vi "Laser_COM.vi"() -> ()   [LabVIEW 2014]
uses:
  <vilib>/Instr/_visa.llb/Select Event Type.ctl
  <vilib>/Instr/_visa.llb/VISA Configure Serial Port (Instr).vi
panel:
  out "Laser":bool
  out "f, kHz":dbl caption="Темп. модуля" format="%#_g kHz"
  out "7":bool
  out "6":bool
  out "4":bool
  out "5":bool
  out "3":bool
  out "2":bool
  out "1":bool
  out "0":bool
  in  "Control PL":bool
  out "DB25 PL":bool
  out "RS232 PL":bool
  out "DB25 GL":bool
  out "RS232 GL":bool
  in  "Control GL":bool
  out "DB25 ML":bool
  out "RS232 ML":bool
  in  "Control ML":bool
  in  "Laser":bool
  out "Laser EM":bool caption="Излучение включено!"
  out "on/off? 3":bool
  out "on/off? 2":bool
  in  "Send":bool
  in  "write buffer":string caption="Передать команду"
  out "COM_connect":bool
  in  "Connect":bool
  out "SN:":string
  out "ID:":string
  out "Guide  laser":bool
  out "module temp":dbl caption="Темп. модуля" format="%#_g °C"
  in  "Power":dbl(slide) caption="Мощность излучения, %" min=0.0 max=100.0 step=0.5 scale=0.0..100.0 scale format="%#.2g"
  in  "Laser pilot":bool caption="Лазер пилот"
  in  "COM":refnum<visa-resource-name>="COM1" caption="Laser COM-port"
  out "read buffer":string caption="ОТВЕТ:"
  out "error out":errorcluster
  in  "error in (no error)":errorcluster
  # "ID:\n\nSN:"
  # "Блок  управления основным лазером"
  # "RS-232"
  # "DB-25"
  # "T модуля -"
  # "RS-232"
  # "Мощьность  излучения, %"
  # "DB-25"
  # "DB-25"
  # "Пилот Лазер"
  # "RS-232"
  # "DB-25"
  # "Терминал"
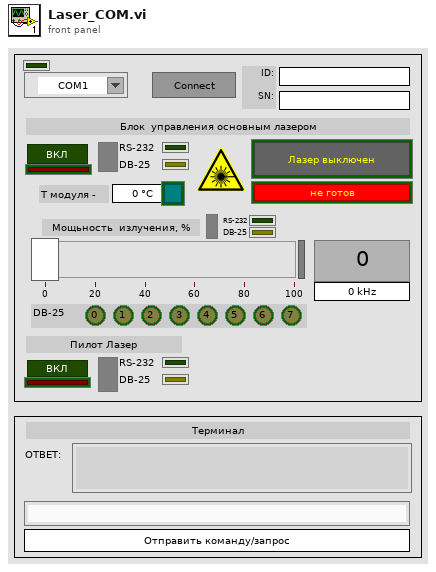
[diagram p1: front panel]
types:
  T1 = typedef "Select Event Type.ctl" = u32
  T2 = cluster{"Power control by DB-25":bool, "Reserved[1]":bool, "AuxOFF control by DB-25":bool, "Guide laser control by DB-25":bool, "Reserved[4]":bool, "Reserved[5]":bool, "Reserved[6]":bool, "Emission Modulation control by DB-25":bool, "The laser is in Jump PRR mode":bool, "Reserved[9]":bool, "Bitstream 1 (BS1) mode is active":bool, "Reserved[11]":bool, "PRR controlled by Sync line in DB-25":bool, "Emission Enable control by DB-25":bool, "APD mode is controlled by DB-25":bool, "Automatic latch":bool, "Reserved[16]":bool, "Reserved[17]":bool, "Reserved[18]":bool, "The laser is in Sweep PRR mode":bool, "The laser is in Follow PRR mode":bool, "Manual Prepump mode is active":bool, "Manual residual is controlled by DB-25":bool, "Reserved[23]":bool, "Reserved[24]":bool, "Guide laser safety function is not activated":bool, "Discharge circuit safety function is activated":bool, "Reserved[27]":bool, "Reserved[28]":bool, "Reserved[29]":bool, "Reserved[30]":bool, "Reserved[31]":bool}
  T3 = cluster{"D0 latched power setting":bool, "D1 latched power setting":bool, "D2 latched power setting":bool, "D3 latched power setting":bool, "D4 latched power setting":bool, "D5 latched power setting":bool, "D6 latched power setting":bool, "D7 latched power setting":bool, "D0 power setting":bool, "D1 power setting":bool, "D2 power setting":bool, "D3 power setting":bool, "D4 power setting":bool, "D5 power setting":bool, "D6 power setting":bool, "D7 power setting":bool, "Latch":bool, "Auxiliary Emission OFF":bool, "Emission Modulation":bool, "Guide laser control":bool, "External Synchronization Input":bool, "Emission enable":bool, "Serial Input":bool, "Serial Clock":bool, "State0":bool, "State1":bool, "State2":bool, "Serial Output":bool, "Serial Enable":bool, "Reserved [29]":bool, "Reserved [30]":bool, "Reserved [31]":bool}
  T4 = cluster{"Rack  reflection":bool, "Temp Laser module":bool, "Temp Laser head":bool, "System Alarm":bool, "+24V main supply Alarm":bool, "HK supply  Alarm":bool, "Laser ready":bool, "Warning is activated":bool}
  T5 = cluster{"Emergency stop":bool, "External PRR [1]":bool, "External PRR [2]":bool, "Reserved [3]":bool, "Reserved [4]":bool, "Guide laser":bool, "Reserved [6]":bool, "Reserved [7]":bool, "Laser emission":bool, "Reserved [9]":bool, "Reserved [10]":bool, "Laser emission command was received by RS-232":bool, "Guide laser command was received by RS-232":bool, "24V Main supply voltage is in specified range":bool, "HK supply voltage is in specified range":bool, "Emission Enable is switched by RS-232":bool, "Reserved [16]":bool, "Reserved [17]":bool, "Reserved [18]":bool, "Reserved [19]":bool, "Reserved [20]":bool, "Reserved [21]":bool, "Reserved [22]":bool, "Reserved [23]":bool, "Reserved [24]":bool, "Reserved [25]":bool, "Reserved [26]":bool, "Reserved [27]":bool, "Reserved [28]":bool, "Reserved [29]":bool, "Reserved [30]":bool, "Reserved [31]":bool}
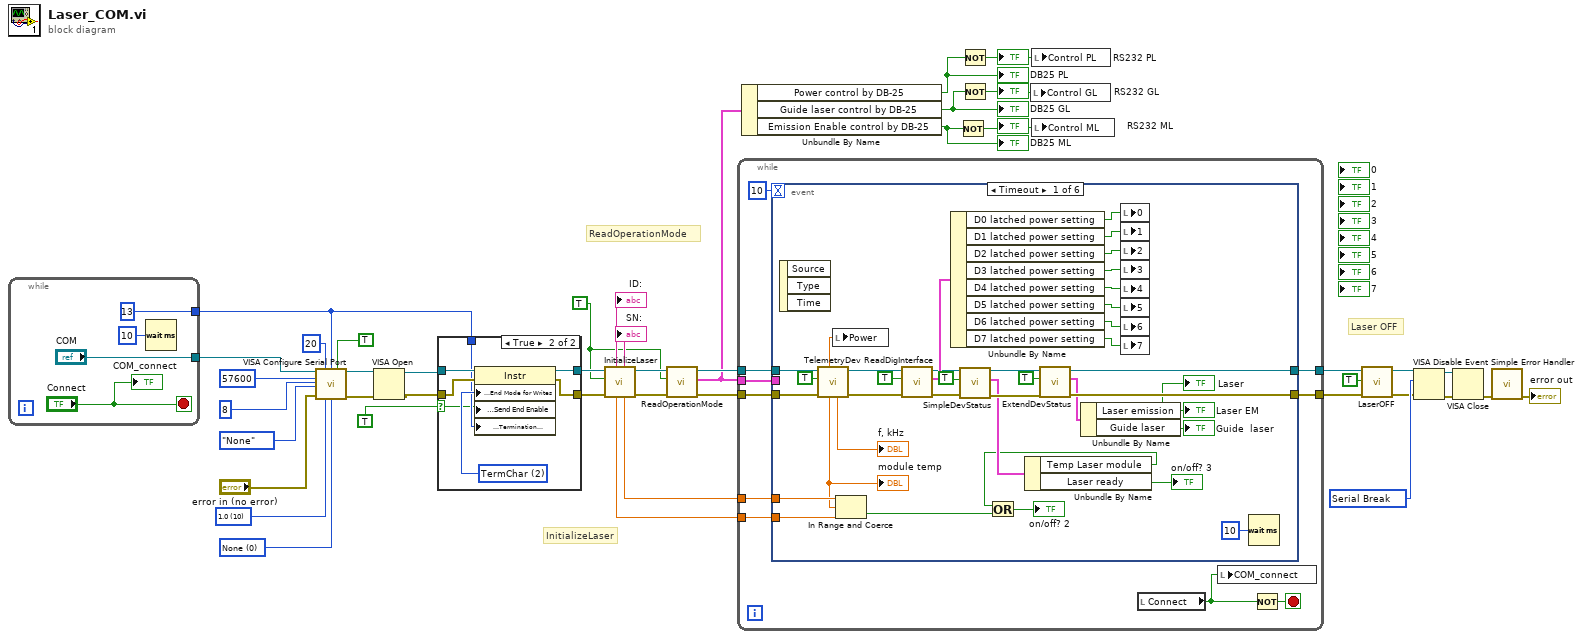
[diagram p0: block diagram]
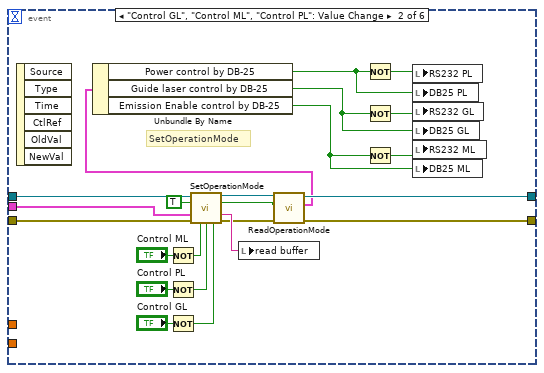
[diagram p2: hidden frame]
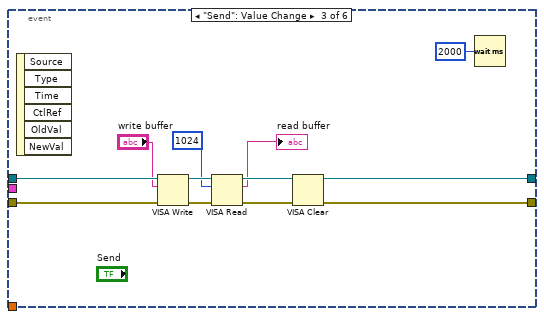
[diagram p3: hidden frame]
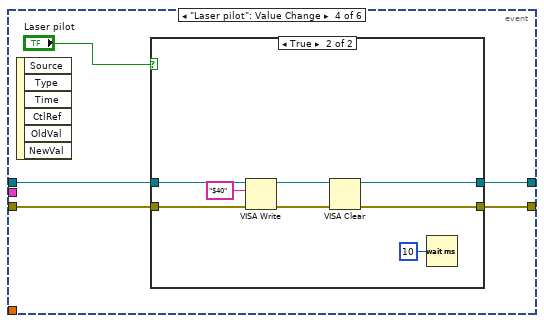
[diagram p4: hidden frame]
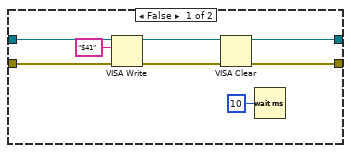
[diagram p5: hidden frame]
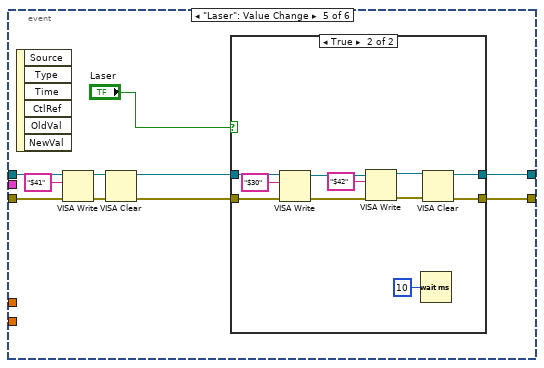
[diagram p6: hidden frame]
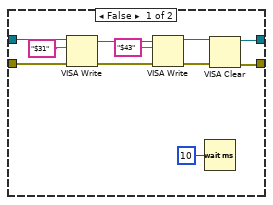
[diagram p7: hidden frame]
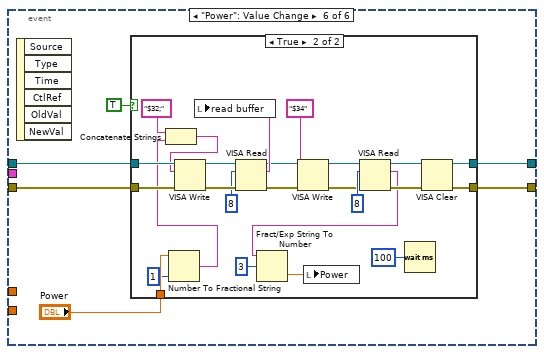
[diagram p8: hidden frame]
diagram:
  w24 = T1 1073684515 items=["Service Request"=1073684491, "Trigger"=3221168138, "Clear"=1073684493, "VXI Signal"=1073684512, "VXI/VME Interrupt"=3221168161, "VXI/VME Sysfail"=1073684509, "VXI/VME Sysreset"=1073684510, "GPIB CIC"=1073684498, "GPIB Talk"=1073684499, "GPIB Listen"=1073684500, "PXI Interrupt"=1073684514, "Serial Break"=1073684515, "Serial TermChar"=1073684516, "Serial CTS"=1073684521, "Serial DSR"=1073684522, "Serial DCD"=1073684524, "Serial RI"=1073684526, "Serial Character"=1073684533, "USB Interrupt"=1073684535, "All Enabled"=1073709055] ("Event Type")
  w29 = u16 0 items=["None", "XON/XOFF", "RTS/CTS", "XON/XOFF & RTS/CTS", "DTR/DSR", "XON/XOFF & DTR/DSR"] ("flow control (0:none)")
  w10 = TRUE
  w36 = u16 10 items=["1.0"=10, "1.5"=15, "2.0"=20] ("stop bits (10: 1 bit)")
  # "Laser OFF"
  # "ReadOperationMode"
  # "InitializeLaser"
  n1 = while {
    tunnel: ["COM"] -> w28
    tunnel: [i16 13 ("term_char")] -> w27
    stop <- "Connect" stop-if-true
    n2 = Wait (ms)(milliseconds to wait=u32 10) -> ()  [unwired: 1 out]
    "COM_connect" <- "Connect"
  }
  n3 = call-poly "VISA Configure Serial Port"("VISA resource name"=w28, "timeout (10sec)"=u32 20, "termination char\n(0xA = '\\n' = LF)"=w27, "Enable Termination\nChar (T)"=TRUE ("Enable Termination\nChar (T)"), "baud rate (9600)"=u32 57600 ("baud rate"), "data bits (8)"=u16 8, "parity (0:none)"=enum16{"None", "Odd", "Even", "Mark", "Space"}."None", "error in (no error)"="error in (no error)", "stop bits (10: 1 bit)"=w36, "flow control (0:none)"=w29) -> ("VISA resource name out"=w39:refnum<visa-resource-name>, "error out"=w38:errorcluster)  [unwired: 4 in]
  n4 = VISA Open(error in (no error)=w38, VISA resource name=w39) -> (VISA resource name=w33:refnum<visa-resource-name>, error out=w34:errorcluster)  [unwired: 3 in]
  n5 = case shown="True" TRUE ("End write with termination character?") {
    selector: TRUE ("End write with termination character?") -> [_ w50]
    tunnel: w33 -> [w48 w56]
    tunnel: w34 -> [w49 w55]
    tunnel: [w48 w54] -> w22
    tunnel: [w49 w53] -> w23
    tunnel: w27 -> [_ w51]
    frame False {
    }
    frame True {
      w52 = u16 2 items=["None", "LastBit", "TermChar", "Break"] ("Serial Settings:Serial End Mode for Writes")
      n6 = property class="Instr"(reference=w56, error in=w55, "Serial Settings:End Mode for Writes"=w52, "Message Based Settings:Send End Enable"=w50, "Message Based Settings:Termination Character"=w51) -> (reference out=w54:refnum<visa-resource-name>, error out=w53:errorcluster)
    }
  }
  n7 = call "InitializeLaser.vi"("error in"=w23, "ON/OFF"=w10, "VISA resource name in"=w22) -> ("error out"=w11:errorcluster, "VISA resource name out"=w12:refnum<visa-resource-name>, "Tmax"=w21:dbl, "SN:"=→"SN:":string, "Tmin"=w20:dbl, "Лазер: ID:"=→"ID:":string)  [unwired: 3 in]
  n8 = call "ReadOperationMode.vi"("error in"=w11, "ON/OFF"=w10, "VISA resource name in"=w12) -> ("error out"=w13:errorcluster, "Operation Mode Status"=w5:T2, "VISA resource name out"=w14:refnum<visa-resource-name>)  [unwired: 5 in, 1 out]
  n9 = while {
    tunnel: w13 -> [w61]
    tunnel: w14 -> [w62]
    tunnel: [w64] -> w16
    tunnel: [w63] -> w15
    tunnel: w21 -> [w59]
    tunnel: w20 -> [w58]
    tunnel: w5 -> [w57]
    stop <- w66 stop-if-true
    n10 = event shown="[0] Timeout" {
      selector: _ -> [_ _ _ _ _ _]
      dyn-events: _ -> [_ _ _ _ _ _]
      timeout: 10 -> [_ _ _ _ _ _]
      tunnel: w62 -> [w96 w125 w137 w142 w167 w196]
      tunnel: w61 -> [w95 w124 w136 w141 w166 w195]
      tunnel: [w100 w112 w131 w140 w164 w194] -> w64
      tunnel: [w99 w113 w130 w139 w163 w193] -> w63
      tunnel: w58 -> [w101 _ _ _ _ _]
      tunnel: w59 -> [w102 _ _ _ _ _]
      tunnel: w57 -> [_ w122 _ _ _ _]
      event Timeout {
        n11 = event-data() -> ()  [unwired: 1 in, 3 out]
        n12 = call "TelemetryDev.vi"("error in"=w95, "ON/OFF"=TRUE, "VISA resource name in"=w96) -> ("error out"=w89:errorcluster, "VISA resource name out"=w90:refnum<visa-resource-name>, "Laser PRR, kHz"=→"f, kHz":dbl, "module temp"=w93:dbl, "Laser Power,%"=w91:dbl)  [unwired: 4 in]
        "module temp" <- w93
        n13 = local write "Power"(w91) -> ()
        n14 = In Range and Coerce(upper limit=w102, x=w93, lower limit=w101) -> (In Range?=w70:bool)  [unwired: 1 out]
        n15 = call "ReadDigInterface.vi"("error in"=w89, "ON/OFF"=TRUE, "VISA resource name in"=w90) -> ("error out"=w77:errorcluster, "Extend Device Status"=w78:T3, "VISA resource name out"=w75:refnum<visa-resource-name>)  [unwired: 5 in]
        n16 = Unbundle By Name(w78) -> ("D0 latched power setting"=w87:bool, "D1 latched power setting"=w86:bool, "D2 latched power setting"=w85:bool, "D3 latched power setting"=w84:bool, "D4 latched power setting"=w83:bool, "D5 latched power setting"=w82:bool, "D6 latched power setting"=w80:bool, "D7 latched power setting"=w81:bool)
        n17 = call "SimpleDevStatus.vi"("error in"=w77, "ON/OFF"=TRUE, "VISA resource name in"=w75) -> ("error out"=w76:errorcluster, "Device Status"=w72:T4, "VISA resource name out"=w74:refnum<visa-resource-name>)  [unwired: 5 in]
        n18 = Unbundle By Name(w72) -> ("Temp Laser module"=w68:bool, "Laser ready"=→"on/off? 3":bool)
        n19 = Or(x=w68, y=w70) -> (x .or. y?=→"on/off? 2":bool)
        n20 = call "ExtendDevStatus.vi"("error in"=w76, "ON/OFF"=TRUE, "VISA resource name in"=w74) -> ("error out"=w99:errorcluster, "Extend Device Status"=w97:T5, "VISA resource name out"=w100:refnum<visa-resource-name>)  [unwired: 5 in]
        n21 = Unbundle By Name(w97) -> ("Laser emission"=→"Laser EM" →"Laser":bool, "Guide laser"=→"Guide  laser":bool)
        n22 = local write "0"(w87) -> ()
        n23 = local write "1"(w86) -> ()
        n24 = local write "2"(w85) -> ()
        n25 = local write "3"(w84) -> ()
        n26 = local write "4"(w83) -> ()
        n27 = local write "5"(w82) -> ()
        n28 = local write "6"(w80) -> ()
        n29 = local write "7"(w81) -> ()
        n30 = Wait (ms)(milliseconds to wait=u32 10) -> ()  [unwired: 1 out]
      }
      event "Control GL", "Control ML", "Control PL": Value Change {
        w110 = TRUE ("ON/OFF")
        # "SetOperationMode"
        n31 = event-data() -> ()  [unwired: 1 in, 6 out]
        n32 = Not(x="Control ML") -> (.not. x?=w117:bool)
        n33 = Not(x="Control PL") -> (.not. x?=w116:bool)
        n34 = Not(x="Control GL") -> (.not. x?=w120:bool)
        n35 = call "SetOperationMode.vi"("VISA resource name in"=w125, "ON/OFF"=w110, "Operation Mode Status"=w122, "error in"=w124, "Laser"=w117, "Power"=w116, "Guide laser"=w120) -> ("VISA resource name out"=w115:refnum<visa-resource-name>, "Message"=w123:string, "error out"=w114:errorcluster)  [unwired: 6 in]
        n36 = local write "read buffer"(w123) -> ()
        n37 = call "ReadOperationMode.vi"("error in"=w114, "ON/OFF"=w110, "VISA resource name in"=w115) -> ("error out"=w113:errorcluster, "Operation Mode Status"=w111:T2, "VISA resource name out"=w112:refnum<visa-resource-name>)  [unwired: 5 in, 1 out]
        n38 = Unbundle By Name(w111) -> ("Power control by DB-25"=w106:bool, "Guide laser control by DB-25"=w105:bool, "Emission Enable control by DB-25"=w104:bool)
        n39 = Not(x=w106) -> (.not. x?=w109:bool)
        n40 = Not(x=w105) -> (.not. x?=w108:bool)
        n41 = Not(x=w104) -> (.not. x?=w107:bool)
        n42 = local write "RS232 PL"(w109) -> ()
        n43 = local write "DB25 PL"(w106) -> ()
        n44 = local write "RS232 GL"(w108) -> ()
        n45 = local write "DB25 GL"(w105) -> ()
        n46 = local write "RS232 ML"(w107) -> ()
        n47 = local write "DB25 ML"(w104) -> ()
      }
      event "Send": Value Change {
        n48 = event-data() -> ()  [unwired: 1 in, 6 out]
        n49 = VISA Write(VISA resource name=w137, write buffer="write buffer", error in (no error)=w136) -> (VISA resource name out=w135:refnum<visa-resource-name>, error out=w134:errorcluster)  [unwired: 1 out]
        n50 = VISA Read(VISA resource name=w135, byte count=u32 1024, error in (no error)=w134) -> (VISA resource name out=w133:refnum<visa-resource-name>, read buffer=→"read buffer":string, error out=w132:errorcluster)  [unwired: 1 out]
        n51 = VISA Clear(VISA resource name=w133, error in (no error)=w132) -> (VISA resource name out=w131:refnum<visa-resource-name>, error out=w130:errorcluster)
        n52 = Wait (ms)(milliseconds to wait=u32 2000) -> ()  [unwired: 1 out]
      }
      event "Laser pilot": Value Change {
        n53 = event-data() -> ()  [unwired: 1 in, 6 out]
        n54 = case shown="True" "Laser pilot" {
          tunnel: w142 -> [w150 w158]
          tunnel: w141 -> [w149 w157]
          tunnel: [w146 w154] -> w140
          tunnel: [w145 w153] -> w139
          frame False {
            n55 = VISA Write(VISA resource name=w150, write buffer="$41", error in (no error)=w149) -> (VISA resource name out=w144:refnum<visa-resource-name>, error out=w143:errorcluster)  [unwired: 1 out]
            n56 = VISA Clear(VISA resource name=w144, error in (no error)=w143) -> (VISA resource name out=w146:refnum<visa-resource-name>, error out=w145:errorcluster)
            n57 = Wait (ms)(milliseconds to wait=u32 10 ("millisecond multiple")) -> ()  [unwired: 1 out]
          }
          frame True {
            n58 = VISA Write(VISA resource name=w158, write buffer="$40", error in (no error)=w157) -> (VISA resource name out=w152:refnum<visa-resource-name>, error out=w151:errorcluster)  [unwired: 1 out]
            n59 = VISA Clear(VISA resource name=w152, error in (no error)=w151) -> (VISA resource name out=w154:refnum<visa-resource-name>, error out=w153:errorcluster)
            n60 = Wait (ms)(milliseconds to wait=u32 10 ("millisecond multiple")) -> ()  [unwired: 1 out]
          }
        }
      }
      event "Laser": Value Change {
        n61 = event-data() -> ()  [unwired: 1 in, 6 out]
        n62 = VISA Write(VISA resource name=w167, write buffer="$41", error in (no error)=w166) -> (VISA resource name out=w162:refnum<visa-resource-name>, error out=w161:errorcluster)  [unwired: 1 out]
        n63 = VISA Clear(VISA resource name=w162, error in (no error)=w161) -> (VISA resource name out=w160:refnum<visa-resource-name>, error out=w159:errorcluster)
        n64 = case shown="True" "Laser" {
          tunnel: w160 -> [w170 w189]
          tunnel: w159 -> [w169 w188]
          tunnel: [w172 w187] -> w164
          tunnel: [w171 w186] -> w163
          frame False {
            n65 = VISA Write(VISA resource name=w170, write buffer="$31", error in (no error)=w169) -> (VISA resource name out=w174:refnum<visa-resource-name>, error out=w173:errorcluster)  [unwired: 1 out]
            n66 = VISA Write(VISA resource name=w174, write buffer="$43", error in (no error)=w173) -> (VISA resource name out=w176:refnum<visa-resource-name>, error out=w175:errorcluster)  [unwired: 1 out]
            n67 = Wait (ms)(milliseconds to wait=u32 10) -> ()  [unwired: 1 out]
            n68 = VISA Clear(VISA resource name=w176, error in (no error)=w175) -> (VISA resource name out=w172:refnum<visa-resource-name>, error out=w171:errorcluster)
          }
          frame True {
            n69 = VISA Write(VISA resource name=w189, write buffer="$30", error in (no error)=w188) -> (VISA resource name out=w181:refnum<visa-resource-name>, error out=w180:errorcluster)  [unwired: 1 out]
            n70 = VISA Write(VISA resource name=w181, write buffer="$42", error in (no error)=w180) -> (VISA resource name out=w183:refnum<visa-resource-name>, error out=w182:errorcluster)  [unwired: 1 out]
            n71 = Wait (ms)(milliseconds to wait=u32 10) -> ()  [unwired: 1 out]
            n72 = VISA Clear(VISA resource name=w183, error in (no error)=w182) -> (VISA resource name out=w187:refnum<visa-resource-name>, error out=w186:errorcluster)
          }
        }
      }
      event "Power": Value Change {
        n73 = event-data() -> ()  [unwired: 1 in, 6 out]
        n74 = case shown="True" TRUE {
          tunnel: w196 -> [w198 w221]
          tunnel: w195 -> [w197 w220]
          tunnel: [w198 w202] -> w194
          tunnel: [w197 w201] -> w193
          tunnel: "Power" -> [_ w217]
          frame False {
          }
          frame True {
            n75 = Number To Fractional String(number=w217, precision (6)=i16 1) -> (F-format string=w212:string)  [unwired: 2 in]
            n76 = Concatenate Strings("$32;" ("write buffer"), w212) -> (w218:string)
            n77 = VISA Write(VISA resource name=w221, write buffer=w218, error in (no error)=w220) -> (VISA resource name out=w223:refnum<visa-resource-name>, error out=w222:errorcluster)  [unwired: 1 out]
            n78 = VISA Read(VISA resource name=w223, byte count=u32 8, error in (no error)=w222) -> (VISA resource name out=w200:refnum<visa-resource-name>, read buffer=w214:string, error out=w199:errorcluster)  [unwired: 1 out]
            n79 = local write "read buffer"(w214) -> ()
            n80 = VISA Write(VISA resource name=w200, write buffer="$34", error in (no error)=w199) -> (VISA resource name out=w205:refnum<visa-resource-name>, error out=w204:errorcluster)  [unwired: 1 out]
            n81 = VISA Read(VISA resource name=w205, byte count=u32 8, error in (no error)=w204) -> (VISA resource name out=w207:refnum<visa-resource-name>, read buffer=w203:string, error out=w208:errorcluster)  [unwired: 1 out]
            n82 = Fract/Exp String To Number(string=w203, offset=3) -> (number=w211:dbl)  [unwired: 2 in, 1 out]
            n83 = local write "Power"(w211) -> ()
            n84 = Wait (ms)(milliseconds to wait=u32 100) -> ()  [unwired: 1 out]
            n85 = VISA Clear(VISA resource name=w207, error in (no error)=w208) -> (VISA resource name out=w202:refnum<visa-resource-name>, error out=w201:errorcluster)
          }
        }
      }
    }
    n86 = local read "Connect"() -> (w65:bool)
    n87 = local write "COM_connect"(w65) -> ()
    n88 = Not(x=w65) -> (.not. x?=w66:bool)
  }
  n89 = Unbundle By Name(w5) -> ("Power control by DB-25"=w1:bool, "Guide laser control by DB-25"=w8:bool, "Emission Enable control by DB-25"=w2:bool)
  "DB25 GL" <- w8
  "DB25 PL" <- w1
  "DB25 ML" <- w2
  n90 = Not(x=w2) -> (.not. x?=w6:bool)
  "RS232 ML" <- w6
  n91 = Not(x=w1) -> (.not. x?=w9:bool)
  "RS232 PL" <- w9
  n92 = Not(x=w8) -> (.not. x?=w7:bool)
  "RS232 GL" <- w7
  n93 = local write "Control GL"(w7) -> ()
  n94 = local write "Control PL"(w9) -> ()
  n95 = local write "Control ML"(w6) -> ()
  n96 = call "LaserOFF.vi"("error in"=w15, "ON/OFF"=TRUE, "VISA resource name in"=w16) -> ("error out"=w3:errorcluster, "VISA resource name out"=w4:refnum<visa-resource-name>)  [unwired: 7 in]
  n97 = VISA Disable Event(8:w3, 10:w24, 11:w4) -> (0:w25:errorcluster, 3:w26:refnum<visa-resource-name>)  [unwired: 1 out]
  n98 = VISA Close(VISA resource name=w26, error in (no error)=w25) -> (error out=w30:errorcluster)
  n99 = call <vilib>:"Simple Error Handler.vi"("error in (no error)"=w30) -> ("error out"=→"error out":errorcluster)  [unwired: 4 in, 4 out]
